vi "HOST.vi"() -> ()   [LabVIEW 2018]
uses:
  <vilib>/userdefined/High Color/nirio_resource_hc.ctl
  <instrlib>/niDCPower/nidcpower.llb/niDCPower Measurement Type.ctl
  <vilib>/FPGAPlugInAG/PXI-7953R/niLvFpga_Open_PXI-7953R.vi
  <vilib>/rvi/interface/common/dynamic/niFpgaDynamicAddResources.vi
  <vilib>/FPGAPlugInAG/Dynamic/niLvFpga_Reset_Dynamic.vi
  <vilib>/FPGAPlugInAG/Dynamic/niLvFpga_Run_Dynamic.vi
  <vilib>/Utility/error.llb/Error Cluster From Error Code.vi
  <vilib>/rvi/errors/niLvFpgaAdjustHostInterfaceError.vi
  <vilib>/rvi/interface/nirviOpenFPGA/nirviOpenFPGA.xnode
  FPGA Bitfiles/DISPLAY_FPGATarget_TARGET_C-Jtn0AUaas.lvbitx
  <vilib>/rvi/interface/nirviMethod/nirviMethod.xnode
  <vilib>/rvi/interface/nirviReadWriteControl/nirviReadWriteControl.xnode
  NiFpgaLv.dll
  <vilib>/rvi/interface/Simulation/niFpgaSimulationCallBeginRW.vi
  <vilib>/FPGAPlugInAG/Dynamic/niLvFpga_WriteFifo_Dynamic.vi
  <vilib>/rvi/errors/niLvFpgaMergeErrorWithErrorCode.vi
panel:
  out "READ_DATA":bool[][](array[boolean])
  in  "WRITE":u8[](array[numeric])=[0, 3, 0, 6, 6, 0, 92, 0, 42, 0, 0, 0]
  in  "R(T)/W(F)":bool
  in  "SEL_Time, мс":u32=100
  out "3V3":bool
  out "VAN":bool
  out "VCC":bool
  out "3V3":u16
  out "VAN":u16
  out "VCC":u16
  in  "3V3_selcur":dbl=0.09 caption="current limit" format="%_6p"
  in  "VAN_selcur":dbl=0.09 caption="current limit" format="%_6p"
  in  "VCC_selcur":dbl=0.09 caption="current limit" format="%_6p"
  out "Image":T1(plugin-control)
  in  "Питание":bool
  out "3V3_char":dbl(graph)=-0.007202656860577676
  out "3V3_cur":dbl caption="measurement" format="%_6g"
  in  "3V3_curlim":dbl=0.1 caption="current limit" format="%_6p"
  in  "3V3, V":dbl=3.3 caption="voltage level" format="%_6p"
  out "VAN_char":dbl(graph)=-0.007202656860577676
  out "VAN_cur":dbl caption="measurement" format="%_6g"
  in  "VAN_curlim":dbl=0.1 caption="current limit" format="%_6p"
  in  "VAN, V":dbl=5.0 caption="voltage level" format="%_6p"
  out "VCC_char":dbl(graph)=-0.007202656860577676
  out "VCC_cur":dbl caption="measurement" format="%_6g"
  in  "VCC_curlim":dbl=0.1 caption="current limit" format="%_6p"
  in  "VCC, V":dbl=1.8 caption="voltage level" format="%_6p"
  out "Частота, Гц":dbl
  in  "Шьем!":bool
  in  "RESET":bool
  in  "ENABLE":bool
  in  "BI":bool
  in  "SERADD":bool
  in  "Темп?":bool
  in  "39":u16=39
  in  "30":u16=30
  in  "20":u16=20
  in  "39":u16=39
  in  "1332":u16=1332
  in  "40":u16=40
  in  "1036":u16=1036
  in  "1550":u16=1550
  in  "Линейки":bool
  in  "0":refnum<k15>="PXI1Slot2"
  in  "1":refnum<k15>="PXI1Slot3"
  in  "FPGA":T2="RIO0"
  in  "LOGS":path=path "C:/VPL/LabView_PRJ/DISPLAY/LOGS"
  out "Номер образца":string="0"
  out "Температура":string="0"
  in  "Картинку передать":bool
  in  "Стоп":bool
  out "Array":u32[][](array[numeric])
  in  "File Path":path=path "C:/Users/Vladislav/Desktop/DISPLAY/DISPLAY/FRAME.bmp"
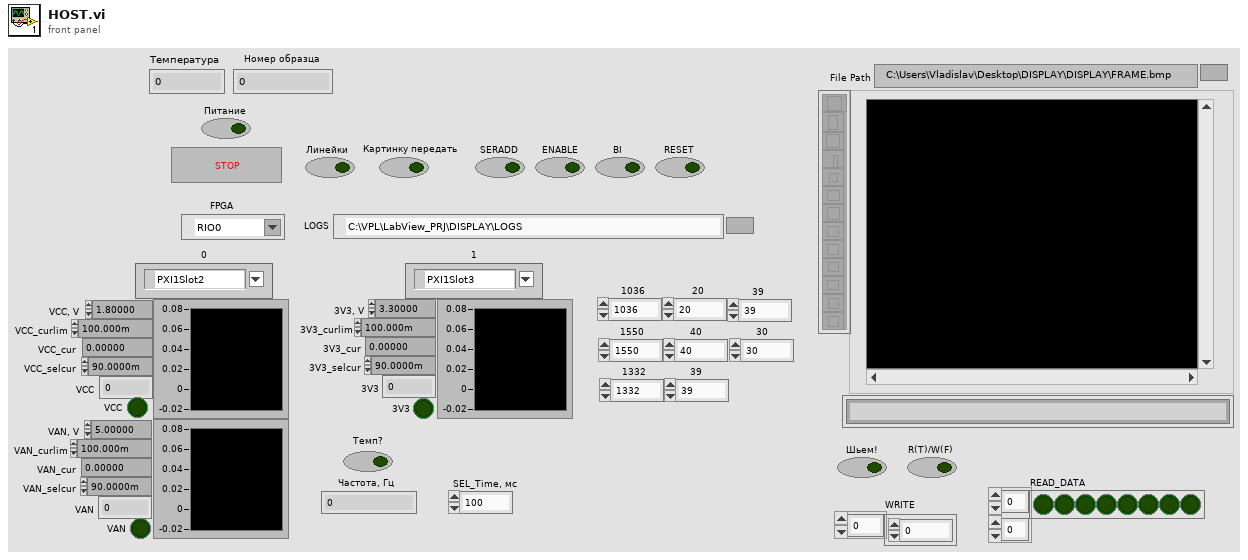
[diagram p1: front panel]
types:
  T1 = typedef "IMAQ Image.ctl" = refnum<image>
  T2 = typedef "nirio_resource_hc.ctl" = tag
  T3 = enum16{"open", "replace", "create", "open or create", "replace or create", "replace or create with confirmation"}
  T4 = typedef "Image Type" = u32
  T5 = typedef "niDCPower Measurement Type.ctl" = i32
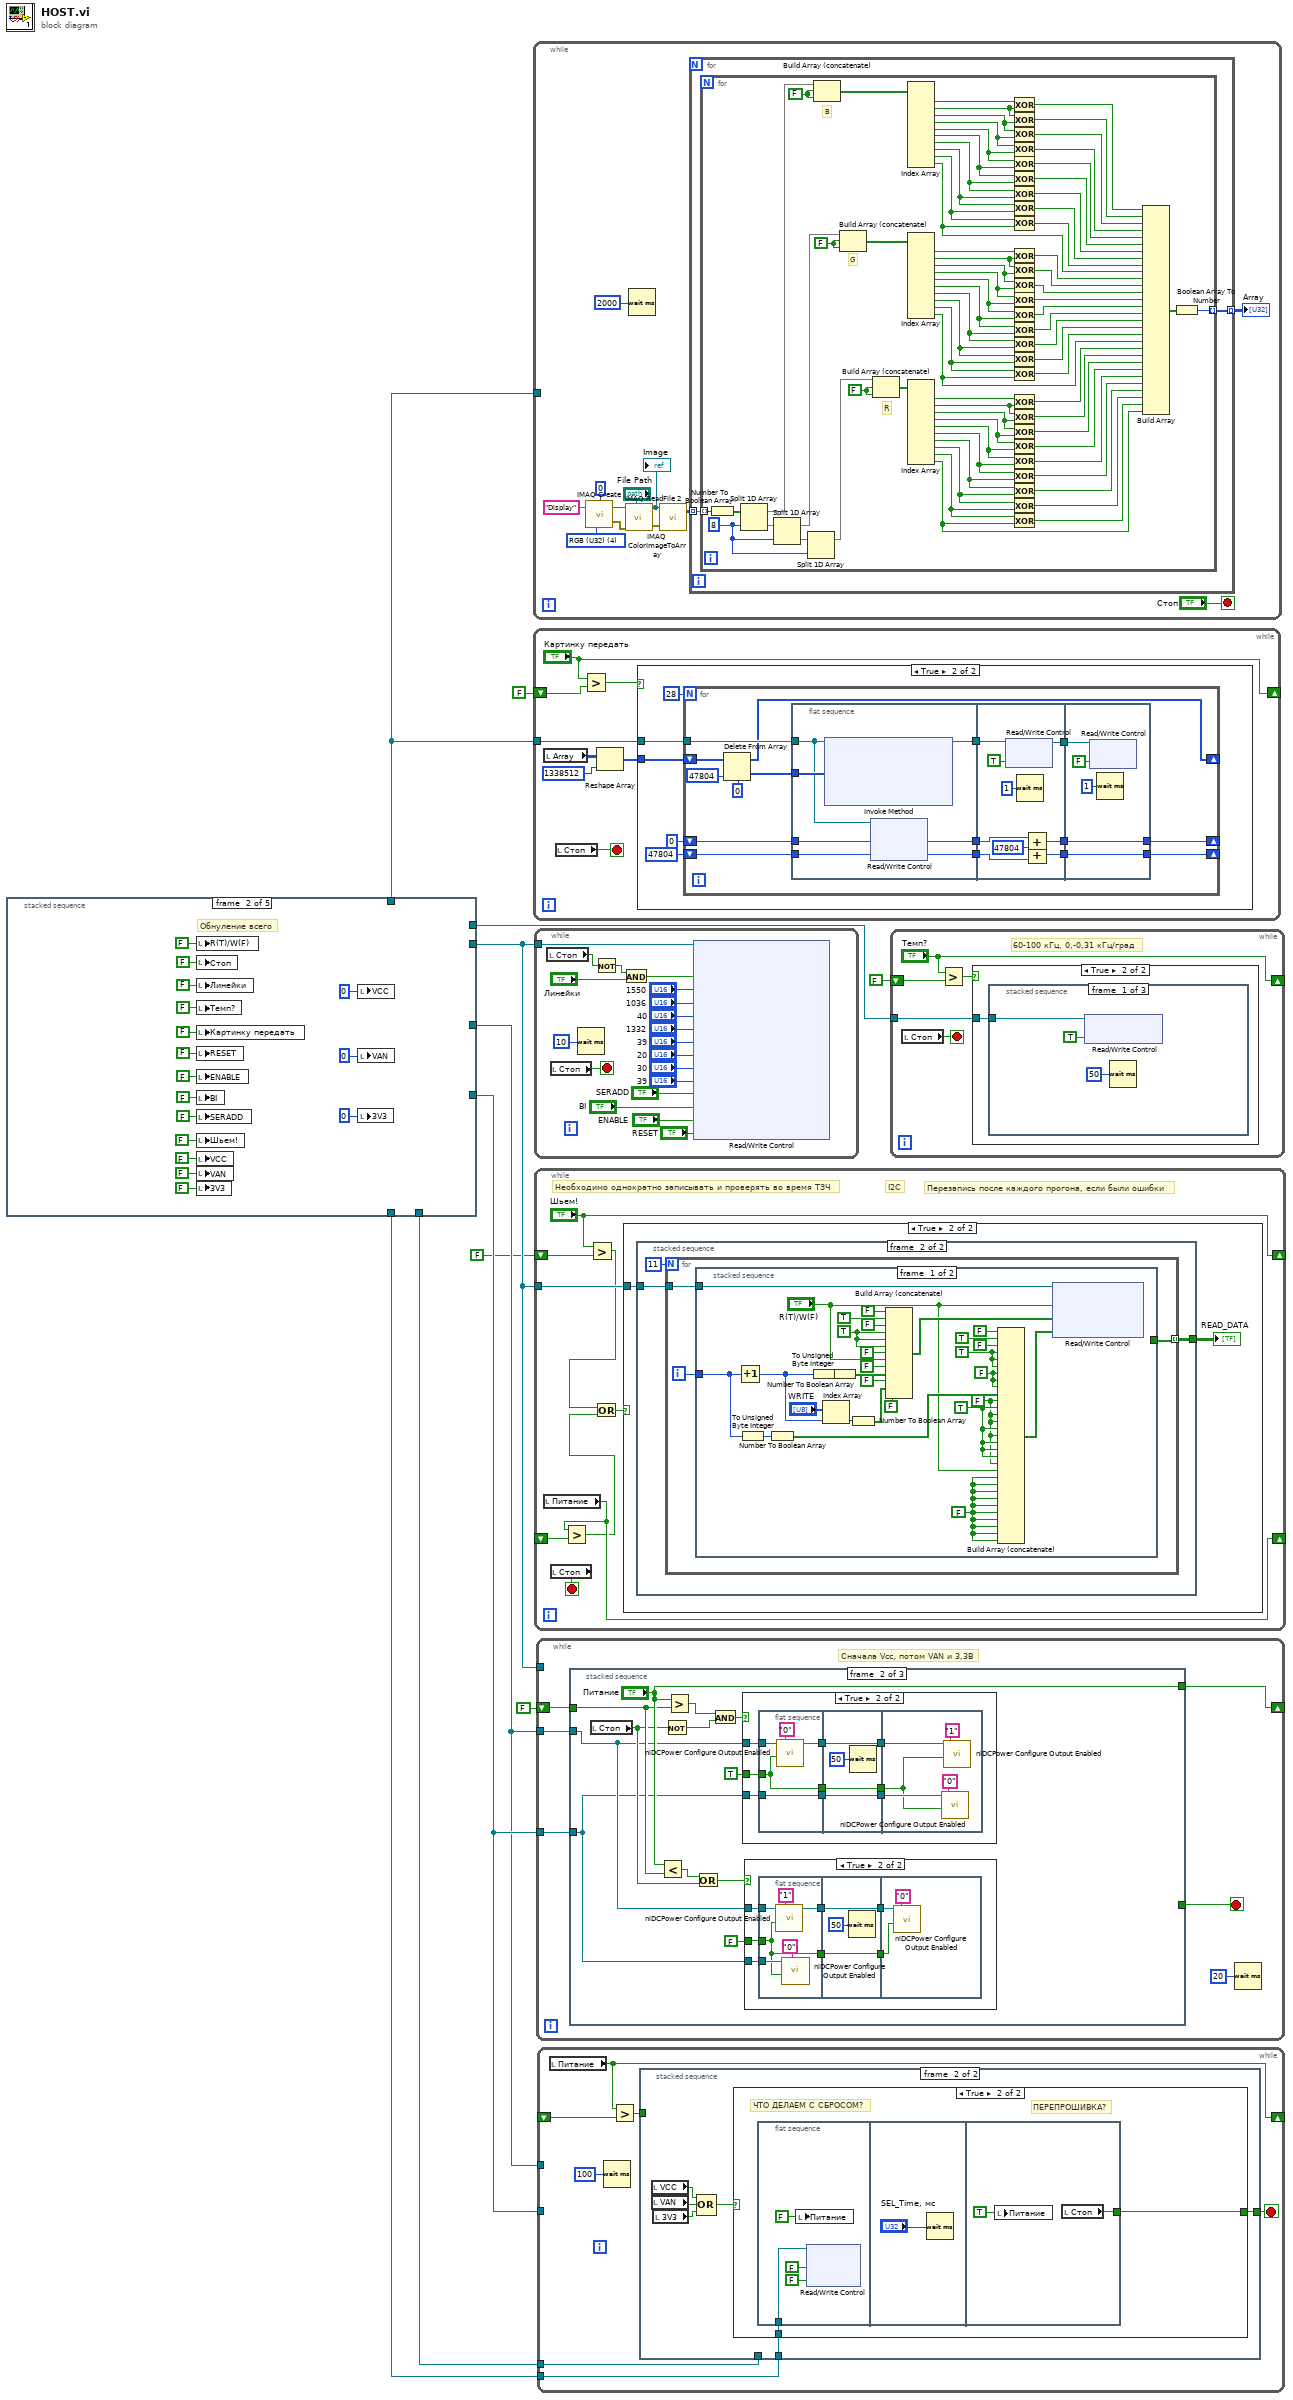
[diagram p0: block diagram]
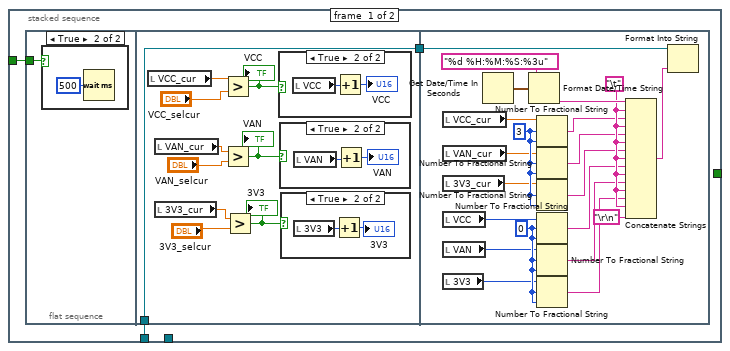
[diagram p2: hidden frame]
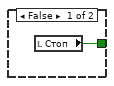
[diagram p7: hidden frame]
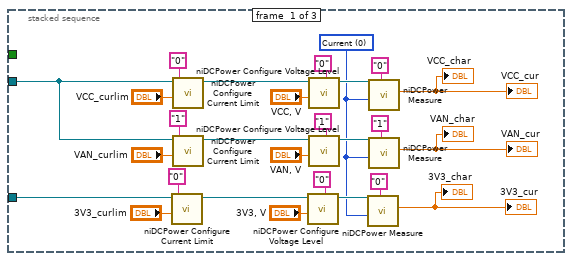
[diagram p8: hidden frame]
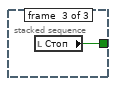
[diagram p11: hidden frame]
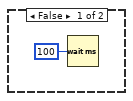
[diagram p12: hidden frame]
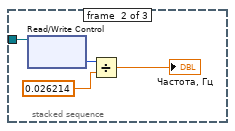
[diagram p13: hidden frame]
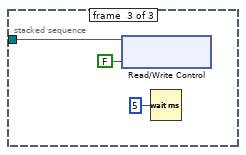
[diagram p14: hidden frame]
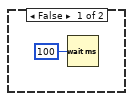
[diagram p15: hidden frame]
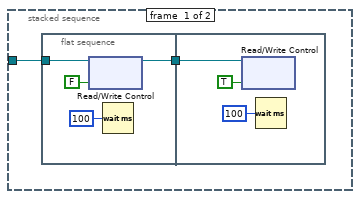
[diagram p16: hidden frame]
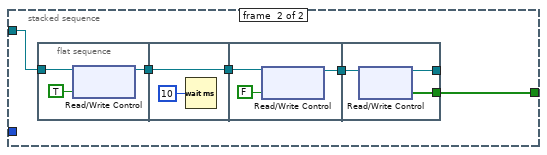
[diagram p17: hidden frame]
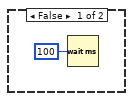
[diagram p18: hidden frame]
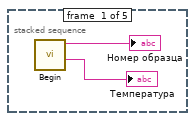
[diagram p19: hidden frame]
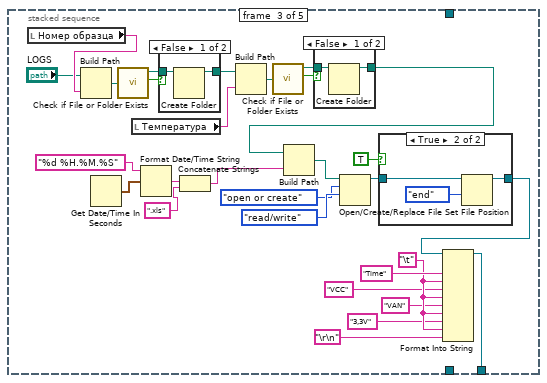
[diagram p20: hidden frame]
diagram:
  n1 = stacked-sequence {
    tunnel: [_ _ _ w69 _] -> w7
    tunnel: [_ _ _ _ w78] -> w2
    tunnel: [_ _ _ _ w77] -> w3
    tunnel: [_ _ _ w69 _] -> w11
    tunnel: [_ _ _ w69 _] -> w5
    tunnel: [_ _ w41 _ _] -> w4
    tunnel: [_ _ _ w69 _] -> w8
    frame #0 {
      n2 = call "Begin.vi"() -> ("Температура 2"=→"Температура":string, "Номер образца 2"=→"Номер образца":string)  [unwired: 10 in]
    }
    frame #1 {
      # "Обнуление всего"
      n3 = local write "R(T)/W(F)"(FALSE ("R(T)/W(F)")) -> ()
      n4 = local write "Стоп"(FALSE ("Стоп")) -> ()
      n5 = local write "Линейки"(FALSE ("Линейки")) -> ()
      n6 = local write "Темп?"(FALSE ("Темп?")) -> ()
      n7 = local write "Картинку передать"(FALSE ("Картинку передать")) -> ()
      n8 = local write "RESET"(FALSE ("RESET")) -> ()
      n9 = local write "ENABLE"(FALSE ("ENABLE")) -> ()
      n10 = local write "BI"(FALSE ("BI")) -> ()
      n11 = local write "SERADD"(FALSE ("SERADD")) -> ()
      n12 = local write "Шьем!"(FALSE ("Шьем!")) -> ()
      n13 = local write "VCC"(FALSE ("VCC")) -> ()
      n14 = local write "VAN"(FALSE ("VAN")) -> ()
      n15 = local write "3V3"(FALSE ("3V3")) -> ()
      n16 = local write "VCC"(u16 0 ("VCC")) -> ()
      n17 = local write "VAN"(u16 0 ("VAN")) -> ()
      n18 = local write "3V3"(u16 0 ("3V3")) -> ()
    }
    frame #2 {
      w34 = "\t"
      n19 = local read "Номер образца"() -> (w58:string)
      n20 = Build Path(base path="LOGS", name or relative path=w58) -> (appended path=w55:path)
      n21 = Get Date/Time In Seconds() -> (seconds since 1Jan1904=w52:timestamp)
      n22 = call <vilib>:"Check if File or Folder Exists.vi"("path"=w55) -> ("file or folder exists?"=w56:bool, "dup path"=w57:path)  [unwired: 8 in, 1 out]
      n23 = local read "Температура"() -> (w36:string)
      n24 = Format Date/Time String(time format string (%c)="%d %H.%M.%S", seconds (now)=w52) -> (date/time string=w50:string)  [unwired: 1 in]
      n25 = case shown="False" w56 {
        tunnel: w57 -> [w67 w68]
        tunnel: [w66 w68] -> w37
        frame False {
          n26 = Create Folder(path (use dialog)=w67) -> (created path=w66:path)  [unwired: 2 in, 2 out]
        }
        frame True {
        }
      }
      n27 = Concatenate Strings(w50, ".xls" ("string")) -> (w49:string)
      n28 = Build Path(base path=w37, name or relative path=w36) -> (appended path=w40:path)
      n29 = call <vilib>:"Check if File or Folder Exists.vi"("path"=w40) -> ("file or folder exists?"=w39:bool, "dup path"=w38:path)  [unwired: 8 in, 1 out]
      n30 = case shown="False" w39 {
        tunnel: w38 -> [w60 w61]
        tunnel: [w59 w61] -> w35
        frame False {
          n31 = Create Folder(path (use dialog)=w60) -> (created path=w59:path)  [unwired: 2 in, 2 out]
        }
        frame True {
        }
      }
      n32 = Build Path(base path=w35, name or relative path=w49) -> (appended path=w51:path)
      n33 = Open/Create/Replace File(file path (use dialog)=w51, operation (0:open)=T3."open or create", access (0:read/write)=enum16{"read/write", "read-only", "write-only"}."read/write") -> (refnum out=w53:refnum<file>)  [unwired: 3 in, 2 out]
      n34 = case shown="True" TRUE {
        tunnel: w53 -> [w62 w65]
        tunnel: [w62 w63] -> w48
        frame False {
        }
        frame True {
          n35 = Set File Position(refnum=w65, from (0:start)=enum16{"start", "end", "current"}."end") -> (refnum out=w63:refnum<file>)  [unwired: 2 in, 1 out]
        }
      }
      n36 = Format Into String(initial string=w48, "Time" ("input 1"), w34, "VCC" ("input 3"), w34, "VAN" ("input 5"), w34, "3,3V" ("input 7"), w34, "\r\n") -> (resulting string=w41:refnum<file>)  [unwired: 2 in, 1 out]
    }
    frame #3 {
      n37 = xnode "Open FPGA VI Reference"("resource name"="FPGA") -> ("FPGA VI Reference Out"=w71:refnum<k20>, "error out"=w73:errorcluster)  [unwired: 1 in]
      n38 = xnode "Invoke Method"("FPGA VI Reference In"=w71, "error in"=w73) -> ("FPGA VI Reference Out"=w74:refnum<k20>, "error out"=w72:errorcluster)
      n39 = xnode "Invoke Method"("FPGA VI Reference In"=w74, "error in"=w72) -> ("FPGA VI Reference Out"=w69:refnum<k20>)  [unwired: 1 in, 1 out]
    }
    frame #4 {
      n40 = call <instrlib>:"niDCPower Initialize.vi"("resource name"="1") -> ("error out"=w81:errorcluster, "instrument handle out"=w79:refnum<k15>)  [unwired: 3 in, 6 out]
      n41 = call <instrlib>:"niDCPower Initialize.vi"("resource name"="0") -> ("error out"=w82:errorcluster, "instrument handle out"=w80:refnum<k15>)  [unwired: 3 in, 6 out]
      n42 = call <instrlib>:"niDCPower Configure Voltage Level.vi"("error in (no error)"=w81, "voltage level"=0.0, "channel name"="0", "instrument handle"=w79) -> ("instrument handle out"=w77:refnum<k15>)  [unwired: 6 in, 1 out]
      n43 = call <instrlib>:"niDCPower Configure Voltage Level.vi"("error in (no error)"=w82, "voltage level"=0.0, "channel name"="0,1", "instrument handle"=w80) -> ("instrument handle out"=w78:refnum<k15>)  [unwired: 6 in, 1 out]
    }
  }
  n44 = while {
    tunnel: w11 -> [_]
    stop <- "Стоп" stop-if-true
    w92 = T4 4 items=["Grayscale (U8)", "Grayscale (I16)", "Grayscale (SGL)", "Complex (CSG)", "RGB (U32)", "HSL (U32)", "RGB (U64)", "Grayscale (U16)"] ("Image Type")
    n45 = call "IMAQ Create"("Border Size"=0, "Image Name"="Display", "Image Type"=w92) -> ("New Image"=w96:T1, "error out"=w93:errorcluster)  [unwired: 2 in]
    n46 = call "IMAQ ReadFile 2"("File Path"="File Path", "error in (no error)"=w93, "Image"=w96) -> ("error out"=w94:errorcluster, "Image Out"=w87:T1)  [unwired: 4 in, 3 out]
    "Image" <- w87
    n47 = Wait (ms)(milliseconds to wait=u32 2000) -> ()  [unwired: 1 out]
    n48 = call "IMAQ ColorImageToArray"("Image"=w87, "error in (no error)"=w94) -> ("Image Pixels (U32)"=w91:u32[][])  [unwired: 2 in, 2 out]
    n49 = for {
      tunnel: w91 -> [w100] mode=indexing
      tunnel: [w99] -> w90 mode=indexing
      n50 = for {
        tunnel: w100 -> [w173] mode=indexing
        tunnel: [w101] -> w99 mode=indexing
        w165 = FALSE
        w166 = FALSE
        w167 = FALSE
        w169 = 8 ("index")
        # "B"
        # "G"
        # "R"
        n51 = Number To Boolean Array(number=w173) -> (Boolean array=w172:bool[])
        n52 = Split 1D Array(array=w172, index=w169) -> (first subarray=w168:bool[], second subarray=w171:bool[])
        n53 = Split 1D Array(array=w171, index=w169) -> (first subarray=w164:bool[], second subarray=w170:bool[])
        n54 = Split 1D Array(array=w170, index=w169) -> (first subarray=w163:bool[])  [unwired: 1 out]
        n55 = Build Array (concatenate)(w168, w167, w167) -> (w162:bool[])
        n56 = Build Array (concatenate)(w164, w166, w166) -> (w143:bool[])
        n57 = Build Array (concatenate)(w163, w165, w165) -> (w133:bool[])
        n58 = Index Array(array=w162) -> (element #1=w161:bool, element #2=w160:bool, element #3=w159:bool, element #4=w158:bool, element #5=w157:bool, element #6=w156:bool, element #7=w155:bool, element #8=w154:bool, element #9=w153:bool, element #10=w123:bool)  [unwired: 10 in]
        n59 = Index Array(array=w143) -> (element #1=w144:bool, element #2=w145:bool, element #3=w146:bool, element #4=w147:bool, element #5=w148:bool, element #6=w149:bool, element #7=w150:bool, element #8=w151:bool, element #9=w152:bool, element #10=w113:bool)  [unwired: 10 in]
        n60 = Index Array(array=w133) -> (element #1=w142:bool, element #2=w141:bool, element #3=w140:bool, element #4=w139:bool, element #5=w138:bool, element #6=w137:bool, element #7=w136:bool, element #8=w135:bool, element #9=w134:bool, element #10=w103:bool)  [unwired: 10 in]
        n61 = Compound Arithmetic op=XOR(w161, w160) -> (w132:bool)
        n62 = Compound Arithmetic op=XOR(w160, w159) -> (w131:bool)
        n63 = Compound Arithmetic op=XOR(w159, w158) -> (w130:bool)
        n64 = Compound Arithmetic op=XOR(w158, w157) -> (w129:bool)
        n65 = Compound Arithmetic op=XOR(w157, w156) -> (w128:bool)
        n66 = Compound Arithmetic op=XOR(w156, w155) -> (w127:bool)
        n67 = Compound Arithmetic op=XOR(w155, w154) -> (w126:bool)
        n68 = Compound Arithmetic op=XOR(w154, w153) -> (w125:bool)
        n69 = Compound Arithmetic op=XOR(w153, w123) -> (w124:bool)
        n70 = Compound Arithmetic op=XOR(w144, w145) -> (w122:bool)
        n71 = Compound Arithmetic op=XOR(w145, w146) -> (w121:bool)
        n72 = Compound Arithmetic op=XOR(w146, w147) -> (w120:bool)
        n73 = Compound Arithmetic op=XOR(w147, w148) -> (w119:bool)
        n74 = Compound Arithmetic op=XOR(w148, w149) -> (w118:bool)
        n75 = Compound Arithmetic op=XOR(w149, w150) -> (w117:bool)
        n76 = Compound Arithmetic op=XOR(w150, w151) -> (w116:bool)
        n77 = Compound Arithmetic op=XOR(w151, w152) -> (w115:bool)
        n78 = Compound Arithmetic op=XOR(w152, w113) -> (w114:bool)
        n79 = Compound Arithmetic op=XOR(w142, w141) -> (w112:bool)
        n80 = Compound Arithmetic op=XOR(w141, w140) -> (w111:bool)
        n81 = Compound Arithmetic op=XOR(w140, w139) -> (w110:bool)
        n82 = Compound Arithmetic op=XOR(w139, w138) -> (w109:bool)
        n83 = Compound Arithmetic op=XOR(w138, w137) -> (w108:bool)
        n84 = Compound Arithmetic op=XOR(w137, w136) -> (w107:bool)
        n85 = Compound Arithmetic op=XOR(w136, w135) -> (w106:bool)
        n86 = Compound Arithmetic op=XOR(w135, w134) -> (w105:bool)
        n87 = Compound Arithmetic op=XOR(w134, w103) -> (w104:bool)
        n88 = Build Array(w132, w131, w130, w129, w128, w127, w126, w125, w124, w123, w122, w121, w120, w119, w118, w117, w116, w115, w114, w113, w112, w111, w110, w109, w108, w107, w106, w105, w104, w103) -> (w102:bool[])
        n89 = Boolean Array To Number(Boolean array=w102) -> (number=w101:u32)
      }
    }
    "Array" <- w90
  }
  n90 = while {
    shift-right: ["Картинку передать"] -> _
    shift-left: FALSE ("Картинку передать") -> [w180]
    tunnel: w11 -> [w177]
    stop <- w181 stop-if-true
    n91 = local read "Array"() -> (w176:u32[][])
    n92 = local read "Стоп"() -> (w181:bool)
    n93 = Greater?(x="Картинку передать", y=w180) -> (0:w178:bool)
    n94 = Reshape Array(w176, 1338512 ("dimension size")) -> (w174:u32[])
    n95 = case shown="True" w178 {
      tunnel: w177 -> [_ w187]
      tunnel: w174 -> [_ w185]
      frame False {
        n96 = Wait (ms)(milliseconds to wait=u32 100) -> ()  [unwired: 1 out]
      }
      frame True {
        n97 = for {
          N: 28 -> [_]
          tunnel: w187 -> [w203]
          shift-right: [w201] -> _
          shift-left: w185 -> [w202]
          shift-right: [w194] -> _
          shift-left: u32 0 -> [w196]
          shift-right: [w191] -> _
          shift-left: u32 47804 -> [w195]
          n98 = Delete From Array(array=w202, length=47804 ("index"), index=0) -> (deleted portion=w198:u32[], array with subset deleted=w201:u32[])
          n99 = flat-sequence {
            tunnel: w203 -> [w206]
            tunnel: w198 -> [w208]
            tunnel: [w207] -> w197
            tunnel: w196 -> [w205]
            tunnel: w195 -> [w204]
            tunnel: [w205] -> w193
            tunnel: [w204] -> w192
            tunnel: w197 -> [w212]
            tunnel: w193 -> [w217]
            tunnel: w192 -> [w214]
            tunnel: [w216] -> w190
            tunnel: [w215] -> w189
            tunnel: [w209] -> w188
            tunnel: [w221] -> w191
            tunnel: [w222] -> w194
            tunnel: w190 -> [w222]
            tunnel: w189 -> [w221]
            tunnel: w188 -> [w219]
            frame #0 {
              n100 = xnode "Invoke Method"("FPGA VI Reference In"=w206, "Data"=w208) -> ("FPGA VI Reference Out"=w207:refnum<k20>)  [unwired: 2 in, 2 out]
              n101 = xnode "Read/Write Control"("FPGA VI Reference In"=w206, "Нач.адр."=w205, "Кон.адр."=w204) -> ()  [unwired: 1 in, 2 out]
            }
            frame #1 {
              w213 = u32 47804
              n102 = xnode "Read/Write Control"("FPGA VI Reference In"=w212, "Запись"=TRUE) -> ("FPGA VI Reference Out"=w209:refnum<k20>)  [unwired: 1 in, 1 out]
              n103 = Wait (ms)(milliseconds to wait=u32 1) -> ()  [unwired: 1 out]
              n104 = Add(x=w217, y=w213) -> (x+y=w216:u32)
              n105 = Add(x=w213, y=w214) -> (x+y=w215:u32)
            }
            frame #2 {
              n106 = xnode "Read/Write Control"("FPGA VI Reference In"=w219, "Запись"=FALSE) -> ()  [unwired: 1 in, 2 out]
              n107 = Wait (ms)(milliseconds to wait=u32 1) -> ()  [unwired: 1 out]
            }
          }
        }
      }
    }
  }
  n108 = while {
    tunnel: w7 -> [w240]
    stop <- w241 stop-if-true
    n109 = local read "Стоп"() -> (w223:bool)
    n110 = local read "Стоп"() -> (w241:bool)
    n111 = Wait (ms)(milliseconds to wait=u32 10) -> ()  [unwired: 1 out]
    n112 = Not(x=w223) -> (.not. x?=w224:bool)
    n113 = And(x=w224, y="Линейки") -> (x .and. y?=w225:bool)
    n114 = xnode "Read/Write Control"("FPGA VI Reference In"=w240, "Линейки"=w225, "1550"="1550", "1036"="1036", "40"="40", "1332"="1332", "39"="39", "20"="20", "30"="30", "39"="39", "SERADD"="SERADD", "BI"="BI", "ENABLE"="ENABLE", "RESET"="RESET") -> ()  [unwired: 2 in, 2 out]
  }
  n115 = while {
    tunnel: w7 -> [w247]
    shift-right: ["Шьем!"] -> _
    shift-left: FALSE ("Шьем!") -> [w249]
    shift-right: [w245] -> _
    shift-left: _ -> [w246]
    stop <- w250 stop-if-true
    # "Перезапись после каждого прогона, если были ошибки"
    # "Необходимо однократно записывать и проверять во время ТЗЧ"
    # "I2C"
    n116 = local read "Питание"() -> (w245:bool)
    n117 = local read "Стоп"() -> (w250:bool)
    n118 = Greater?(x=w245, y=w246) -> (0:w242:bool)
    n119 = Greater?(x="Шьем!", y=w249) -> (0:w243:bool)
    n120 = Or(x=w243, y=w242) -> (x .or. y?=w244:bool)
    n121 = case shown="True" w244 {
      tunnel: w247 -> [_ w253]
      frame False {
        n122 = Wait (ms)(milliseconds to wait=u32 100) -> ()  [unwired: 1 out]
      }
      frame True {
        n123 = stacked-sequence {
          tunnel: w253 -> [w255 w265]
          tunnel: [_ w263] -> w252
          frame #0 {
            n124 = flat-sequence {
              tunnel: w255 -> [w259]
              tunnel: [w256] -> w254
              tunnel: w254 -> [w261]
              frame #0 {
                n125 = xnode "Read/Write Control"("FPGA VI Reference In"=w259, "RESET"=FALSE) -> ("FPGA VI Reference Out"=w256:refnum<k20>)  [unwired: 1 in, 1 out]
                n126 = Wait (ms)(milliseconds to wait=u32 100) -> ()  [unwired: 1 out]
              }
              frame #1 {
                n127 = xnode "Read/Write Control"("FPGA VI Reference In"=w261, "RESET"=TRUE) -> ()  [unwired: 1 in, 2 out]
                n128 = Wait (ms)(milliseconds to wait=u32 100) -> ()  [unwired: 1 out]
              }
            }
          }
          frame #1 {
            n129 = for {
              N: 11 -> [_]
              tunnel: w265 -> [w268]
              tunnel: [w266] -> w263 mode=indexing
              i -> [w267]
              n130 = stacked-sequence {
                tunnel: w268 -> [w297 w302]
                tunnel: w267 -> [w274 _]
                tunnel: [_ w298] -> w266
                frame #0 {
                  w269 = FALSE ("element")
                  w271 = TRUE ("element")
                  w270 = FALSE ("element")
                  w276 = FALSE ("element")
                  w286 = TRUE ("element")
                  w291 = TRUE ("element")
                  n131 = Increment(x=w274) -> (x+1=w280:i32)
                  n132 = To Unsigned Byte Integer(number=w274) -> (unsigned 8bit integer=w275:u8)
                  n133 = Number To Boolean Array(number=w275) -> (Boolean array=w273:bool[])
                  n134 = To Unsigned Byte Integer(number=w280) -> (unsigned 8bit integer=w285:u8)
                  n135 = Index Array(array="WRITE", index=w280) -> (element=w278:u8)
                  n136 = Number To Boolean Array(number=w285) -> (Boolean array=w283:bool[])
                  n137 = Number To Boolean Array(number=w278) -> (Boolean array=w277:bool[])
                  n138 = Build Array (concatenate)(FALSE ("element"), TRUE ("element"), FALSE ("element"), w291, w291, w291, FALSE ("element"), "R(T)/W(F)", FALSE ("element"), w283, FALSE ("element"), w277, FALSE ("element")) -> (w296:bool[])
                  n139 = Build Array (concatenate)(FALSE ("element"), TRUE ("element"), FALSE ("element"), w286, w286, w286, w276, w276, w276, w273, w270, w271, w270, w270, w271, w270, w271, w271, w271, w270, "R(T)/W(F)", w269, w269, w269, w269, w269, w269, w269, w269, w269, w269) -> (w295:bool[])
                  n140 = xnode "Read/Write Control"("FPGA VI Reference In"=w297, "R(T)/W(F)"="R(T)/W(F)", "I2C[26:0]_WRITE"=w296, "I2C[37:0]_READ"=w295) -> ()  [unwired: 1 in, 2 out]
                }
                frame #1 {
                  n141 = flat-sequence {
                    tunnel: w302 -> [w305]
                    tunnel: [w303] -> w301
                    tunnel: w301 -> [w306]
                    tunnel: [w306] -> w300
                    tunnel: w300 -> [w310]
                    tunnel: [w308] -> w299
                    tunnel: w299 -> [w313]
                    tunnel: [w312] -> _
                    tunnel: [w311] -> w298
                    frame #0 {
                      n142 = xnode "Read/Write Control"("FPGA VI Reference In"=w305, "Регистр!"=TRUE) -> ("FPGA VI Reference Out"=w303:refnum<k20>)  [unwired: 1 in, 1 out]
                    }
                    frame #1 {
                      n143 = Wait (ms)(milliseconds to wait=u32 10) -> ()  [unwired: 1 out]
                    }
                    frame #2 {
                      n144 = xnode "Read/Write Control"("FPGA VI Reference In"=w310, "Регистр!"=FALSE) -> ("FPGA VI Reference Out"=w308:refnum<k20>)  [unwired: 1 in, 1 out]
                    }
                    frame #3 {
                      n145 = xnode "Read/Write Control"("FPGA VI Reference In"=w313) -> ("FPGA VI Reference Out"=w312:refnum<k20>, "DATA"=w311:bool[])  [unwired: 1 in, 1 out]
                    }
                  }
                }
              }
            }
          }
        }
        "READ_DATA" <- w252
      }
    }
  }
  n146 = while {
    tunnel: w2 -> [w318]
    tunnel: w3 -> [w319]
    tunnel: w7 -> [_]
    shift-right: [w315] -> _
    shift-left: FALSE -> [w316]
    stop <- w317 stop-if-true
    # "Сначала Vcc, потом VAN и 3,3В"
    n147 = stacked-sequence {
      tunnel: w319 -> [w321 w349 _]
      tunnel: w318 -> [w320 w350 _]
      tunnel: [_ _ w401] -> w317
      tunnel: w316 -> [_ w354 _]
      tunnel: [_ "Питание" _] -> w315
      frame #0 {
        w322 = T5 0 items=["Current", "Voltage"] ("measurement type")
        n148 = call <instrlib>:"niDCPower Configure Current Limit.vi"("current limit"="3V3_curlim", "channel name"="0", "instrument handle"=w321) -> ("instrument handle out"=w328:refnum<k15>)  [unwired: 7 in, 1 out]
        n149 = call <instrlib>:"niDCPower Configure Current Limit.vi"("current limit"="VCC_curlim", "channel name"="0", "instrument handle"=w320) -> ("instrument handle out"=w344:refnum<k15>)  [unwired: 7 in, 1 out]
        n150 = call <instrlib>:"niDCPower Configure Current Limit.vi"("current limit"="VAN_curlim", "channel name"="1", "instrument handle"=w320) -> ("instrument handle out"=w333:refnum<k15>)  [unwired: 7 in, 1 out]
        n151 = call <instrlib>:"niDCPower Configure Voltage Level.vi"("voltage level"="3V3, V", "channel name"="0", "instrument handle"=w328) -> ("instrument handle out"=w324:refnum<k15>)  [unwired: 7 in, 1 out]
        n152 = call <instrlib>:"niDCPower Configure Voltage Level.vi"("voltage level"="VCC, V", "channel name"="0", "instrument handle"=w344) -> ("instrument handle out"=w340:refnum<k15>)  [unwired: 7 in, 1 out]
        n153 = call <instrlib>:"niDCPower Configure Voltage Level.vi"("voltage level"="VAN, V", "channel name"="1", "instrument handle"=w333) -> ("instrument handle out"=w337:refnum<k15>)  [unwired: 7 in, 1 out]
        n154 = call <instrlib>:"niDCPower Measure.vi"("measurement type"=w322, "channel name"="0", "instrument handle"=w324) -> ("measurement"=→"3V3_cur" →"3V3_char":dbl)  [unwired: 6 in, 2 out]
        n155 = call <instrlib>:"niDCPower Measure.vi"("measurement type"=w322, "channel name"="0", "instrument handle"=w340) -> ("measurement"=→"VCC_cur" →"VCC_char":dbl)  [unwired: 6 in, 2 out]
        n156 = call <instrlib>:"niDCPower Measure.vi"("measurement type"=w322, "channel name"="1", "instrument handle"=w337) -> ("measurement"=→"VAN_cur" →"VAN_char":dbl)  [unwired: 6 in, 2 out]
      }
      frame #1 {
        n157 = local read "Стоп"() -> (w352:bool)
        n158 = Less?(x="Питание", y=w354) -> (x < y?=w353:bool)
        n159 = Not(x=w352) -> (.not. x?=w358:bool)
        n160 = Greater?(x="Питание", y=w354) -> (0:w356:bool)
        n161 = Or(x=w353, y=w352) -> (x .or. y?=w351:bool)
        n162 = And(x=w356, y=w358) -> (x .and. y?=w357:bool)
        n163 = case shown="True" w357 {
          tunnel: w349 -> [_ w380]
          tunnel: w350 -> [_ w379]
          tunnel: TRUE -> [_ w378]
          frame False {
          }
          frame True {
            n164 = flat-sequence {
              tunnel: [w390] -> w386
              tunnel: w380 -> [w390]
              tunnel: [w389] -> w385
              tunnel: [w387] -> w384
              tunnel: w379 -> [w388]
              tunnel: w378 -> [w387]
              tunnel: [w394] -> w383
              tunnel: w386 -> [w394]
              tunnel: [w393] -> w382
              tunnel: w385 -> [w393]
              tunnel: [w392] -> w381
              tunnel: w384 -> [w392]
              tunnel: w383 -> [w400]
              tunnel: w382 -> [w399]
              tunnel: w381 -> [w396]
              frame #0 {
                n165 = call <instrlib>:"niDCPower Configure Output Enabled.vi"("output enabled"=w387, "channel name"="0", "instrument handle"=w388) -> ("instrument handle out"=w389:refnum<k15>)  [unwired: 7 in, 1 out]
              }
              frame #1 {
                n166 = Wait (ms)(milliseconds to wait=u32 50) -> ()  [unwired: 1 out]
              }
              frame #2 {
                n167 = call <instrlib>:"niDCPower Configure Output Enabled.vi"("output enabled"=w396, "channel name"="0", "instrument handle"=w400) -> ()  [unwired: 7 in, 2 out]
                n168 = call <instrlib>:"niDCPower Configure Output Enabled.vi"("output enabled"=w396, "channel name"="1", "instrument handle"=w399) -> ()  [unwired: 7 in, 2 out]
              }
            }
          }
        }
        n169 = case shown="True" w351 {
          tunnel: w350 -> [_ w361]
          tunnel: w349 -> [_ w360]
          tunnel: FALSE -> [_ w359]
          frame False {
          }
          frame True {
            n170 = flat-sequence {
              tunnel: w360 -> [w367]
              tunnel: [w370] -> w365
              tunnel: [w366] -> w364
              tunnel: w361 -> [w369]
              tunnel: w359 -> [w366]
              tunnel: [w373] -> w363
              tunnel: w365 -> [w373]
              tunnel: [w372] -> w362
              tunnel: w364 -> [w372]
              tunnel: w363 -> [w377]
              tunnel: w362 -> [w375]
              frame #0 {
                n171 = call <instrlib>:"niDCPower Configure Output Enabled.vi"("output enabled"=w366, "channel name"="1", "instrument handle"=w369) -> ("instrument handle out"=w370:refnum<k15>)  [unwired: 7 in, 1 out]
                n172 = call <instrlib>:"niDCPower Configure Output Enabled.vi"("output enabled"=w366, "channel name"="0", "instrument handle"=w367) -> ()  [unwired: 7 in, 2 out]
              }
              frame #1 {
                n173 = Wait (ms)(milliseconds to wait=u32 50) -> ()  [unwired: 1 out]
              }
              frame #2 {
                n174 = call <instrlib>:"niDCPower Configure Output Enabled.vi"("output enabled"=w375, "channel name"="0", "instrument handle"=w377) -> ()  [unwired: 7 in, 2 out]
              }
            }
          }
        }
      }
      frame #2 {
        n175 = local read "Стоп"() -> (w401:bool)
      }
    }
    n176 = Wait (ms)(milliseconds to wait=u32 20) -> ()  [unwired: 1 out]
  }
  n177 = while {
    tunnel: w5 -> [w403]
    tunnel: w4 -> [w404]
    tunnel: w3 -> [_]
    tunnel: w2 -> [_]
    shift-right: [w406] -> _
    shift-left: _ -> [w407]
    stop <- w402 stop-if-true
    n178 = local read "Питание"() -> (w406:bool)
    n179 = Wait (ms)(milliseconds to wait=u32 100) -> ()  [unwired: 1 out]
    n180 = Greater?(x=w406, y=w407) -> (0:w405:bool)
    n181 = stacked-sequence {
      tunnel: w405 -> [w411 _]
      tunnel: w404 -> [w409 _]
      tunnel: w403 -> [_ w452]
      tunnel: [_ w451] -> w402
      frame #0 {
        n182 = flat-sequence {
          tunnel: w411 -> [w412]
          tunnel: [w414] -> w410
          tunnel: w409 -> [w414]
          tunnel: w410 -> [w430]
          frame #0 {
            n183 = case shown="True" w412 {
              frame False {
              }
              frame True {
                n184 = Wait (ms)(milliseconds to wait=u32 500) -> ()  [unwired: 1 out]
              }
            }
          }
          frame #1 {
            n185 = local read "VCC_cur"() -> (w423:dbl)
            n186 = local read "VAN_cur"() -> (w421:dbl)
            n187 = local read "3V3_cur"() -> (w419:dbl)
            n188 = Greater?(x=w423, y="VCC_selcur") -> (0:w417:bool)
            "VCC" <- w417
            n189 = Greater?(x=w421, y="VAN_selcur") -> (0:w416:bool)
            "VAN" <- w416
            n190 = Greater?(x=w419, y="3V3_selcur") -> (0:w415:bool)
            "3V3" <- w415
            n191 = case shown="True" w417 {
              frame False {
              }
              frame True {
                n192 = local read "VCC"() -> (w429:u16)
                n193 = Increment(x=w429) -> (x+1=→"VCC":u16)
              }
            }
            n194 = case shown="True" w416 {
              frame False {
              }
              frame True {
                n195 = local read "VAN"() -> (w427:u16)
                n196 = Increment(x=w427) -> (x+1=→"VAN":u16)
              }
            }
            n197 = case shown="True" w415 {
              frame False {
              }
              frame True {
                n198 = local read "3V3"() -> (w425:u16)
                n199 = Increment(x=w425) -> (x+1=→"3V3":u16)
              }
            }
          }
          frame #2 {
            w444 = "\t"
            w446 = i16 0 ("width (-)")
            w447 = i16 3 ("width (-)")
            n200 = local read "VCC_cur"() -> (w433:dbl)
            n201 = local read "VAN_cur"() -> (w432:dbl)
            n202 = local read "3V3_cur"() -> (w431:dbl)
            n203 = local read "VCC"() -> (w436:u16)
            n204 = local read "VAN"() -> (w435:u16)
            n205 = local read "3V3"() -> (w434:u16)
            n206 = Get Date/Time In Seconds() -> (seconds since 1Jan1904=w450:timestamp)
            n207 = Format Date/Time String(time format string (%c)="%d %H:%M:%S:%3u", seconds (now)=w450) -> (date/time string=w448:string)  [unwired: 1 in]
            n208 = Number To Fractional String(number=w433, width (-)=w447, precision (6)=w447) -> (F-format string=w442:string)  [unwired: 1 in]
            n209 = Number To Fractional String(number=w432, width (-)=w447, precision (6)=w447) -> (F-format string=w441:string)  [unwired: 1 in]
            n210 = Number To Fractional String(number=w431, width (-)=w447, precision (6)=w447) -> (F-format string=w440:string)  [unwired: 1 in]
            n211 = Number To Fractional String(number=w436, width (-)=w446, precision (6)=w446) -> (F-format string=w439:string)  [unwired: 1 in]
            n212 = Number To Fractional String(number=w435, width (-)=w446, precision (6)=w446) -> (F-format string=w438:string)  [unwired: 1 in]
            n213 = Number To Fractional String(number=w434, width (-)=w446, precision (6)=w446) -> (F-format string=w437:string)  [unwired: 1 in]
            n214 = Concatenate Strings(w448, w444, w442, w444, w441, w444, w440, w444, w439, w444, w438, w444, w437, w444, "\r\n") -> (w445:string)
            n215 = Format Into String(initial string=w430, w445) -> ()  [unwired: 2 in, 2 out]
          }
        }
      }
      frame #1 {
        n216 = local read "VCC"() -> (w456:bool)
        n217 = local read "VAN"() -> (w455:bool)
        n218 = local read "3V3"() -> (w454:bool)
        n219 = Compound Arithmetic op=OR(w456, w455, w454) -> (w453:bool)
        n220 = case shown="True" w453 {
          tunnel: w452 -> [_ w459]
          tunnel: [w457 w458] -> w451
          frame False {
            n221 = local read "Стоп"() -> (w457:bool)
          }
          frame True {
            # "ПЕРЕПРОШИВКА?"
            # "ЧТО ДЕЛАЕМ С СБРОСОМ?"
            n222 = flat-sequence {
              tunnel: w459 -> [w463]
              tunnel: [w465] -> w458
              frame #0 {
                n223 = local write "Питание"(FALSE ("Питание")) -> ()
                n224 = xnode "Read/Write Control"("FPGA VI Reference In"=w463, "Линейки"=FALSE, "RESET"=FALSE) -> ()  [unwired: 1 in, 2 out]
              }
              frame #1 {
                n225 = Wait (ms)(milliseconds to wait="SEL_Time, мс") -> ()  [unwired: 1 out]
              }
              frame #2 {
                n226 = local write "Питание"(TRUE ("Питание")) -> ()
                n227 = local read "Стоп"() -> (w465:bool)
              }
            }
          }
        }
      }
    }
  }
  n228 = while {
    shift-right: ["Темп?"] -> _
    shift-left: FALSE ("Темп?") -> [w470]
    tunnel: w8 -> [w467]
    stop <- w471 stop-if-true
    # "60-100 кГц, 0,-0,31 кГц/град"
    n229 = local read "Стоп"() -> (w471:bool)
    n230 = Greater?(x="Темп?", y=w470) -> (0:w468:bool)
    n231 = case shown="True" w468 {
      tunnel: w467 -> [_ w473]
      frame False {
        n232 = Wait (ms)(milliseconds to wait=u32 100) -> ()  [unwired: 1 out]
      }
      frame True {
        n233 = stacked-sequence {
          tunnel: w473 -> [w476 w480 w482]
          frame #0 {
            n234 = xnode "Read/Write Control"("FPGA VI Reference In"=w476, "Температура?"=TRUE) -> ()  [unwired: 1 in, 2 out]
            n235 = Wait (ms)(milliseconds to wait=u32 50) -> ()  [unwired: 1 out]
          }
          frame #1 {
            n236 = xnode "Read/Write Control"("FPGA VI Reference In"=w480) -> ("Фронты"=w479:u16)  [unwired: 1 in, 2 out]
            n237 = Divide(x=w479, y=0.026214) -> (x/y=→"Частота, Гц":dbl)
          }
          frame #2 {
            n238 = xnode "Read/Write Control"("FPGA VI Reference In"=w482, "Температура?"=FALSE) -> ()  [unwired: 1 in, 2 out]
            n239 = Wait (ms)(milliseconds to wait=u32 5) -> ()  [unwired: 1 out]
          }
        }
      }
    }
  }
